vi "ListMFCchannels.vi"(11 "Gas Release System":string) -> (0 "C2H6descriptions":T1[](array[typedef]), 1 "N2descriptions":T1[](array[typedef]), 2 "ValveChannels":string[](array[string]))   [LabVIEW 2016]
uses:
  MFCdescription.ctl
  MFCcapability.ctl
  ADAM Client/Sub VIs/ADAM Controls/Channel_names.ctl
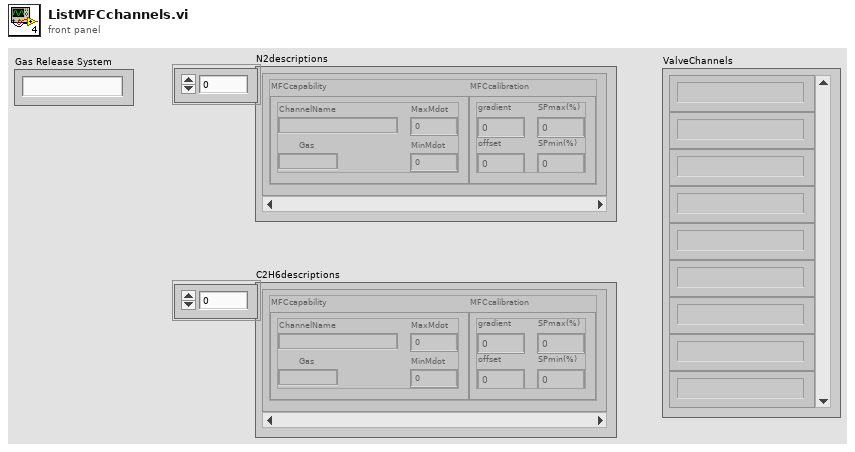
[diagram p1: front panel]
types:
  T1 = typedef "MFCdescription.ctl" = cluster{"MFCcapability":T2, "MFCcalibration":cluster{"gradient":dbl, "offset":dbl, "SPmin(%)":dbl, "SPmax(%)":dbl}}
  T2 = typedef "MFCcapability.ctl" = cluster{"ChannelName":string, "MinMdot":dbl, "MaxMdot":dbl, "Gas":string}
  T3 = typedef "Channel_names.ctl" = enum16{"Active Only", "Active + Off", "All Channels"}
  T4 = typedef "Ch_description_ADAM.ctl" = cluster{"Ch Name":string, "Type":T5, "Function":T6, "Ch State":T7, "Calibration type":T8, "A":dbl, "B":dbl, "C":dbl, "D":dbl, "Comments":string, "Address":T9, "String":string, "Duty":u16}
  T5 = typedef "Module_type_ADAM.ctl" = string
  T6 = typedef "Function_ADAM.ctl" = enum16{"Analogue Input", "Digital Input", "Event counter", "Event rate", "Analogue Output", "Digital Output", "Relay Output"}
  T7 = typedef "Channel_State.ctl" = enum16{"On", "Off", "Always On", "Always Off"}
  T8 = typedef "Calib_type_ADAM.ctl" = string
  T9 = typedef "Address.ctl" = cluster{"Main":i32, "Ch.":i32, "Sub":i32, "Port Name":string}
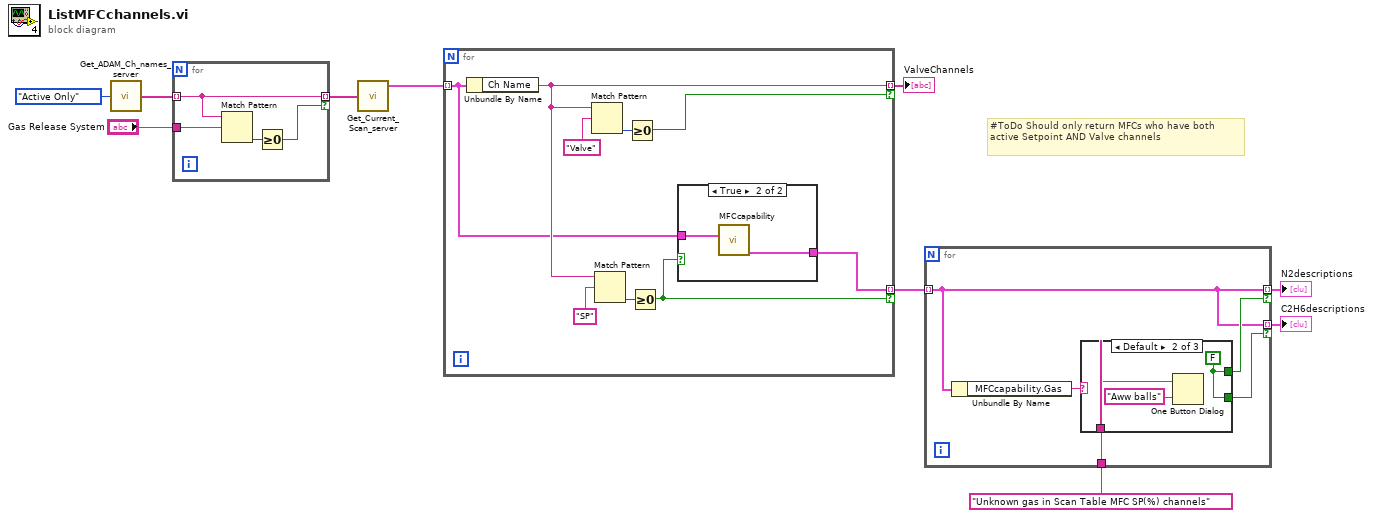
[diagram p0: block diagram]
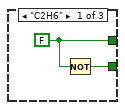
[diagram p2: hidden frame]
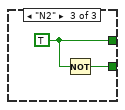
[diagram p3: hidden frame]
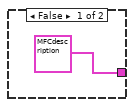
[diagram p4: hidden frame]
diagram:
  # "#ToDo Should only return MFCs who have both active Setpoint AND Valve channels"
  n1 = call "Get_ADAM_Ch_names_server.vi"("Channel names set"=Channel_names."Active Only") -> ("Ch names"=w8:string[])
  n2 = for {
    tunnel: w8 -> [w12] mode=indexing
    tunnel: "Gas Release System" -> [w14]
    tunnel: [w12] -> w10 mode=indexing if=w11
    n3 = Match Pattern(string=w12, regular expression=w14) -> (offset past match=w13:i32)  [unwired: 1 in, 3 out]
    n4 = Greater Or Equal To 0?(x=w13) -> (x >= 0?=w11:bool)
  }
  n5 = call "Get_Current_Scan_server.vi"("Desired Channels"=w10) -> ("Ch Description Array"=w6:T4[])  [unwired: 2 out]
  n6 = for {
    tunnel: w6 -> [w16] mode=indexing
    tunnel: [w18] -> w5 mode=indexing if=w21
    tunnel: [w15] -> w3 mode=indexing if=w17
    n7 = Unbundle By Name(w16) -> ("Ch Name"=w18:string)
    n8 = Match Pattern(string=w18, regular expression="Valve") -> (offset past match=w23:i32)  [unwired: 1 in, 3 out]
    n9 = Match Pattern(string=w18, regular expression="SP") -> (offset past match=w20:i32)  [unwired: 1 in, 3 out]
    n10 = Greater Or Equal To 0?(x=w23) -> (x >= 0?=w21:bool)
    n11 = Greater Or Equal To 0?(x=w20) -> (x >= 0?=w17:bool)
    n12 = case shown="True" w17 {
      tunnel: w16 -> [_ w26]
      tunnel: [T1 {"MFCcapability"={"ChannelName"="GRC-A:C2H6-8:SP(%)", "MinMdot"=1.0, "MaxMdot"=19.0, "Gas"="C2H6"}, "MFCcalibration"={"gradient"=0.0, "offset"=0.0, "SPmin(%)"=0.0, "SPmax(%)"=0.0}} ("MFCdescription") w25] -> w15
      frame False {
      }
      frame True {
        n13 = call "MFCcapability.vi"("Ch Description"=w26) -> ("MFCdescription"=w25:T1)  [unwired: 10 in]
      }
    }
  }
  "ValveChannels" <- w5
  n14 = for {
    tunnel: "Unknown gas in Scan Table MFC SP(%) channels" ("message") -> [w30]
    tunnel: [w27] -> w2 mode=indexing if=w29
    tunnel: [w27] -> w1 mode=indexing if=w28
    tunnel: w3 -> [w27] mode=indexing
    n15 = Unbundle By Name(w27) -> ("MFCcapability.Gas"=w31:string)
    n16 = case shown="Default" w31 {
      tunnel: w30 -> [_ w36 _]
      tunnel: [w33 w34 w38] -> w29
      tunnel: [w32 w34 w37] -> w28
      frame "C2H6" {
        w33 = FALSE
        n17 = Not(x=w33) -> (.not. x?=w32:bool)
      }
      frame Default {
        w34 = FALSE
        n18 = One Button Dialog(message=w36, button name ("OK")="Aww balls") -> ()  [unwired: 1 out]
      }
      frame "N2" {
        w38 = TRUE
        n19 = Not(x=w38) -> (.not. x?=w37:bool)
      }
    }
  }
  "N2descriptions" <- w2
  "C2H6descriptions" <- w1
